vi "Stop Core.vi"(10 "final error code":i32, 11 "IViewable in":refnum<class "IViewable.lvclass">) -> (3 "IViewable out":refnum<class "IViewable.lvclass">)   [LabVIEW 2020, in "MVA Framework.lvlib" / "IViewable.lvlib" / "IViewable.lvclass"]
doc: "(<B>Filename</B>: Actor Framework.lvlib:Actor.lvclass:Stop Core.vi)\n\nDefines what the actor does before it stops. Use the <B>final error code</B> input to determine whether the actor shut down in response to an error.\n\nBy default, this method does nothing. A descendant class may override it to define behavior, such as shutting down any processes the actor initiated in its override of the Actor Core method.\n\n<License>\nCopyright © 2017 Composed Systems, LLC | All rights reserved\nwww.composed.io\n\nAuthor: Ethan Stern <ethan.stern@composed.io>\n\nThis software is provided \"AS IS\" WITHOUT WARRANTIES, either express or implied, AND IS FOR EDUCATIONAL PURPOSES ONLY.\n</License>"
uses:
  IViewable.lvclass
  IViewable.lvclass/IViewable.ctl
  ActorEvents/IEventAggregator/IEventAggregator.lvclass
  mva-core/Source/IObserver/IObserver Messages/Unsubscribe Msg/Unsubscribe Msg.lvclass
  <vilib>/ActorFramework/Actor/Actor.lvclass
  ProtectedSubpanel/ProtectedSubpanel.lvclass
  C:/Program Files/National Instruments/LabVIEW 2020/vi.lib/ActorFramework/Actor/Actor.lvclass
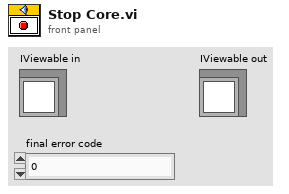
[diagram p1: front panel]
types:
  T1 = typedef "MVA Framework.lvlib/IViewable.lvlib/ProtectedSubpanel.lvclass/Protected Subpanel Reference.ctl" = refnum<data-value>
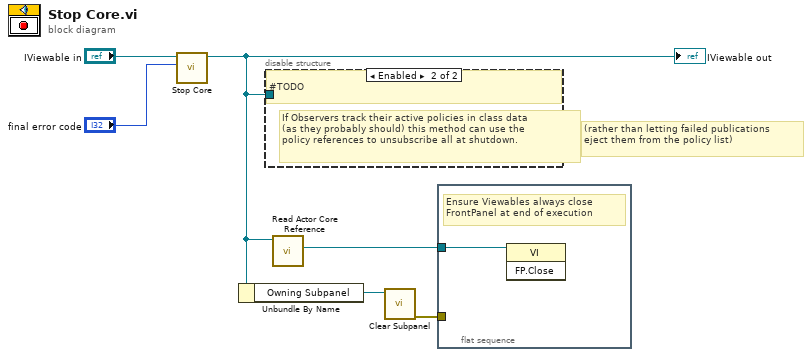
[diagram p0: block diagram]
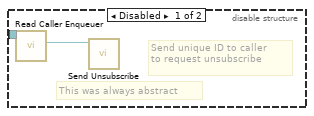
[diagram p2: hidden frame]
diagram:
  # "(rather than letting failed publications\neject them from the policy list)"
  n1 = call-parent "Stop Core.vi"("final error code"="final error code", "IObserver in"="IViewable in") -> ("IObserver out"=w1:refnum<class "IViewable.lvclass">)  [unwired: 9 in]
  "IViewable out" <- w1
  n2 = Unbundle By Name(w1) -> ("Owning Subpanel"=w3:T1)
  n3 = disable-structure shown="Enabled" {
    disable-tunnel: w1 -> [w7 _]
    frame Disabled {
      # "This was always abstract"
      # "Send unique ID to caller\nto request unsubscribe"
      n4 = call <vilib>:"Read Caller Enqueuer.vi"("Actor"=w7) -> ("Caller Enqueuer"=w8:refnum<class "Message Enqueuer.lvclass">)  [unwired: 10 in]
      n5 = call "Send Unsubscribe.vi"("Message Enqueuer"=w8) -> ()  [unwired: 9 in, 2 out]
    }
    frame Enabled {
      # "If Observers track their active policies in class data\n(as they probably should) this method can use the\npolicy references to unsubscribe all at shutdown."
      # "#TODO"
    }
  }
  n6 = call "Read Actor Core Reference.vi"("IViewable In"=w1) -> ("Actor Core Refnum"=w4:refnum<vi>)  [unwired: 9 in, 1 out]
  n7 = call "Clear Subpanel.vi"("Protected Subpanel"=w3) -> ("error out"=w2:errorcluster)  [unwired: 9 in, 1 out]
  n8 = flat-sequence {
    tunnel: w4 -> [w9]
    tunnel: w2 -> [_]
    frame #0 {
      # "Ensure Viewables always close\nFrontPanel at end of execution"
      n9 = invoke class="VI" method="FP.Close"(reference=w9) -> ()  [unwired: 2 in, 3 out]
    }
  }
